vi "Example1b.vi"() -> ()   [LabVIEW 2011]
uses:
  Interprocess Messenger/QueueMessenger/QueueMessenger.lvclass
  Interprocess Messenger/TextVarientMessage/MSG.lvclass
  Interprocess Messenger/TextVarientMessage/Extract Text (static).vi
  Interprocess Messenger/TextVarientMessage/Write (no data).vi
  Interprocess Messenger/Send/Send.lvclass
  Interprocess Messenger/Send/Send Message.vi
  Interprocess Messenger/Send/Send (no data).vi
  Parallel Process/Messsage Logger/Message Logger.lvclass
  Interprocess Messenger/Messenger (Parent)/MGR.lvclass
  Interprocess Messenger/SendOnly/Observer.lvclass
  Messenging.lvlib
  Interprocess Messenger/TextVarientMessage/Reply (varient).vi
  Interprocess Messenger/SendMultiple/Create Observer.vi
  Interprocess Messenger/SendMultiple/ObserverSet.lvclass
panel:
  out "Time":string
  # "Any Key Down to stop"
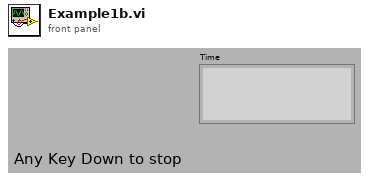
[diagram p1: front panel]
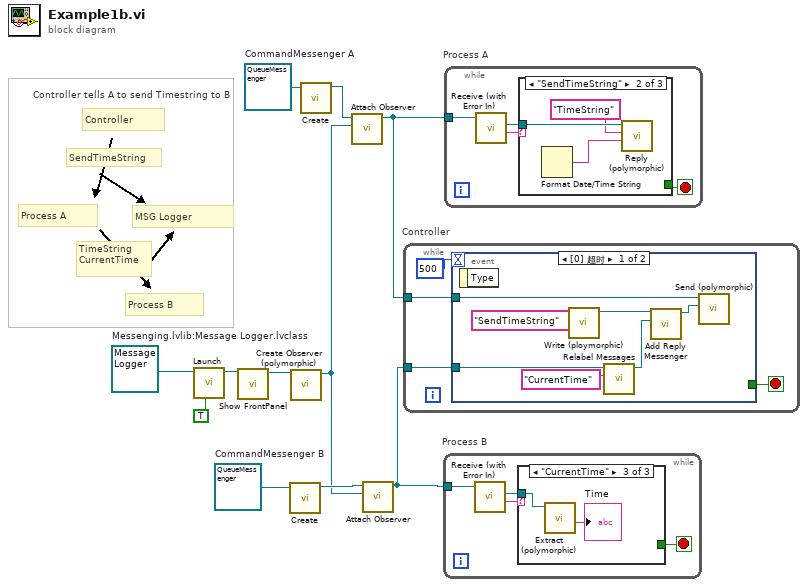
[diagram p0: block diagram]
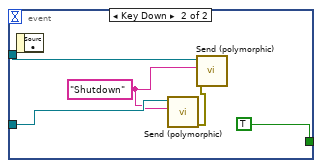
[diagram p2: hidden frame]
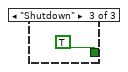
[diagram p4: hidden frame]
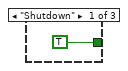
[diagram p5: hidden frame]
diagram:
  w1 = refnum<class "Message Logger.lvclass"> refnum  # Messenging.lvlib:Message Logger.lvclass
  w10 = refnum<class "QueueMessenger.lvclass"> refnum  # CommandMessenger A
  w11 = refnum<class "QueueMessenger.lvclass"> refnum  # CommandMessenger B
  # "MSG Logger"
  # "TimeString \nCurrentTime"
  # "Controller tells A to send Timestring to B"
  # "SendTimeString"
  # "Process B"
  # "Process A"
  # "Controller"
  n1 = call-dynamic "Launch.vi"("AutoShutdown Slave (F)"=TRUE, "Parallel Process in"=w1) -> ("Parallel Process out"=w3:refnum<class "Message Logger.lvclass">)  [unwired: 2 in, 7 out]
  n2 = call-dynamic "Show FrontPanel.vi"("Parallel Process in"=w3) -> ("Parallel Process out"=w4:refnum<class "Message Logger.lvclass">)  [unwired: 2 in, 8 out]
  n3 = call-dynamic "Create.vi"("QueueMessenger in"=w11) -> ("QueueMessenger out"=w9:refnum<class "QueueMessenger.lvclass">)  [unwired: 1 in, 9 out]
  n4 = call-poly "Create Observer (polymorphic).vi"("Input"=w4) -> ("Observer"=w5:refnum<class "Observer.lvclass">)  [unwired: 1 in, 7 out]
  n5 = call-dynamic "Create.vi"("QueueMessenger in"=w10) -> ("QueueMessenger out"=w8:refnum<class "QueueMessenger.lvclass">)  [unwired: 1 in, 9 out]
  n6 = call "Attach Observer.vi"("Observer(s)"=w5, "MGR.lvclass in"=w8) -> ("MGR.lvclass out"=w6:refnum<class "QueueMessenger.lvclass">)  [unwired: 1 in, 8 out]
  n7 = call "Attach Observer.vi"("Observer(s)"=w5, "MGR.lvclass in"=w9) -> ("MGR.lvclass out"=w7:refnum<class "QueueMessenger.lvclass">)  [unwired: 1 in, 8 out]
  n8 = while "Controller" {
    tunnel: w6 -> [w15]
    tunnel: w7 -> [w14]
    stop <- w13 stop-if-true
    n9 = event shown="[0] 超时" {
      selector: _ -> [_ _]
      dyn-events: _ -> [_ _]
      timeout: 500 -> [_ _]
      tunnel: w15 -> [w19 w26]
      tunnel: w14 -> [w18 w24]
      tunnel: [_ TRUE] -> w13
      event Timeout {
        n10 = event-data() -> ()  [unwired: 2 out]
        n11 = call-poly "Write (ploymorphic).vi"("Label"="SendTimeString") -> ("Message"=w21:refnum<class "MSG.lvclass">)  [unwired: 1 in, 9 out]
        n12 = call "Relabel Messages.vi"("Relabel messages with"="CurrentTime" ("Reply Label"), "Send IN"=w18) -> ("Observer"=w17:refnum<class "Observer.lvclass">)  [unwired: 9 out]
        n13 = call "Add Reply Messenger.vi"("Reply to..."=w17, "Message"=w21) -> ("Message"=w22:refnum<class "MSG.lvclass">)  [unwired: 2 in, 7 out]
        n14 = call-poly "Send (polymorphic).vi"("Message"=w22, "MSR Parent in"=w19) -> ()  [unwired: 1 in, 9 out]
      }
      event Key Down {
        w23 = "Shutdown"
        n15 = event-data() -> ()  [unwired: 2 out]
        n16 = call-poly "Send (polymorphic).vi"("Label"=w23, "MSR Parent in"=w24) -> ("error out"=w25:errorcluster)  [unwired: 1 in, 8 out]
        n17 = call-poly "Send (polymorphic).vi"("error in (no error)"=w25, "Label"=w23, "MSR Parent in"=w26) -> ()  [unwired: 9 out]
      }
    }
  }
  n18 = while "Process B" {
    tunnel: w7 -> [w31]
    stop <- w28 stop-if-true
    n19 = call-dynamic "Receive (with Error In).vi"("MGR in"=w31) -> ("Label"=w30:string, "Message"=w29:refnum<class "MSG.lvclass">)  [unwired: 2 in, 7 out]
    n20 = case shown="\"CurrentTime\"" w30 {
      tunnel: w29 -> [_ _ w34]
      tunnel: [TRUE _ _] -> w28
      frame "Shutdown" {
      }
      frame Default {
      }
      frame "CurrentTime" {
        n21 = call-poly "Extract (polymorphic).vi"("TextMessage in"=w34) -> ("Text"=→"Time":string)  [unwired: 1 in, 9 out]
      }
    }
  }
  n22 = while "Process A" {
    tunnel: w6 -> [w38]
    stop <- w35 stop-if-true
    n23 = call-dynamic "Receive (with Error In).vi"("MGR in"=w38) -> ("Label"=w37:string, "Message"=w36:refnum<class "MSG.lvclass">)  [unwired: 2 in, 7 out]
    n24 = case shown="\"SendTimeString\"" w37 {
      tunnel: w36 -> [_ w41 _]
      tunnel: [_ _ TRUE] -> w35
      frame "False", Default {
      }
      frame "SendTimeString" {
        n25 = Format Date/Time String() -> (date/time string=w39:string)  [unwired: 3 out]
        n26 = call-poly "Reply (polymorphic).vi"("Varient"=w39, "Reply"="TimeString", "Message to Reply to"=w41) -> ()  [unwired: 1 in, 8 out]
      }
      frame "Shutdown" {
      }
    }
  }
